vi "WhoInheritsWhom.vi"(0 "reference":refnum<class "ClassRelationshipEdge.lvclass">, 5 "error in (no error)":errorcluster) -> (14 "reference out":refnum<class "ClassRelationshipEdge.lvclass">, 15 "inherits":refnum<class "AbstractNode.lvclass">, 16 "base":refnum<class "AbstractNode.lvclass">, 17 "inheritanceUsed":bool, 19 "error out":errorcluster)   [LabVIEW 2016, in "ClassRelationshipEdge.lvclass"]
doc: "In which direction is the Triangle point, pointing."
uses:
  <resource>/Framework/Providers/Open_GDS/UML/ClassRelationshipEdge_class/ClassRelationshipEdge.lvclass
  C:/Program Files (x86)/National Instruments/LabVIEW 2016/resource/Framework/Providers/Open_GDS/UML/SegmentedLineEdge_class/SegmentedLineEdge.lvclass
  C:/Program Files (x86)/National Instruments/LabVIEW 2016/resource/Framework/Providers/Open_GDS/UML/AbstractEdge_class/AbstractEdge.lvclass
  <resource>/Framework/Providers/Open_GDS/UML/AbstractNode_class/AbstractNode.lvclass
  <resource>/Framework/Providers/Open_GDS/UML/ArrowHead_class/ArrowHead.lvclass
  <resource>/Framework/Providers/Open_GDS/UML/SegmentedLineEdge_class/SegmentedLineEdge.lvclass
  <resource>/Framework/Providers/Open_GDS/UML/AbstractEdge_class/AbstractEdge.lvclass
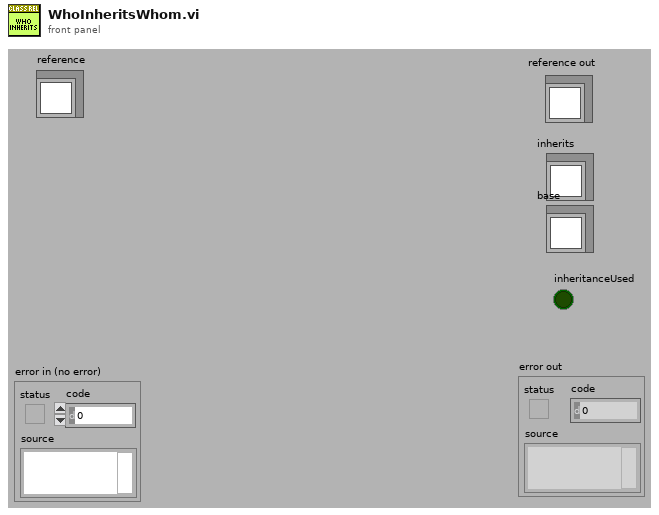
[diagram p1: front panel]
types:
  T1 = typedef "SegmentedLineEdge.lvclass/ObjectAttributes.ctl" = cluster{"lineStyle":refnum<class "LineStyle.lvclass">, "startArrowHead":refnum<class "ArrowHead.lvclass">, "endArrowHead":refnum<class "ArrowHead.lvclass">, "startLabel":string, "midLabel":string, "endLabel":string, "MidLabelOffset":T2, "SplitWire":bool}
  T2 = typedef "Point Point2D.ctl" = cluster{"x":dbl, "y":dbl}
  T3 = typedef "AbstractEdge.lvclass/ObjectAttributes.ctl" = cluster{"start":refnum<class "AbstractNode.lvclass">, "end":refnum<class "AbstractNode.lvclass">}
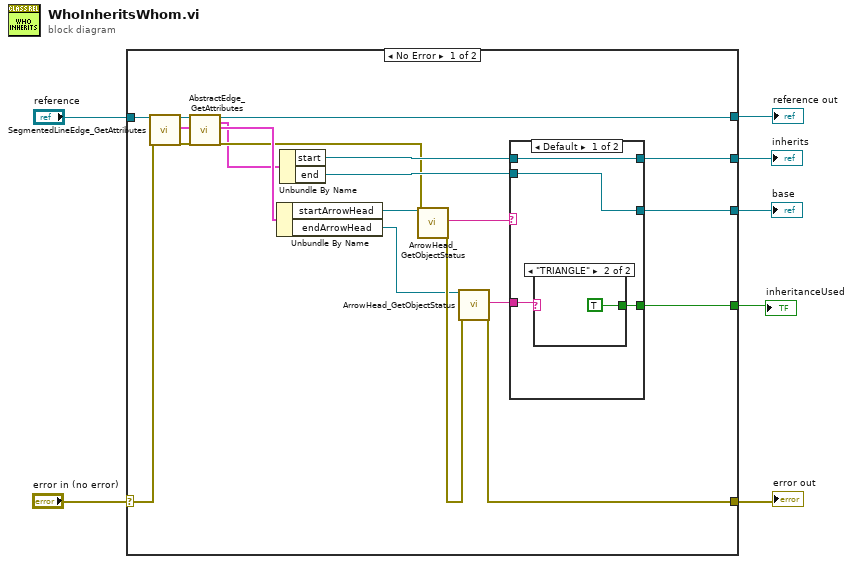
[diagram p0: block diagram]
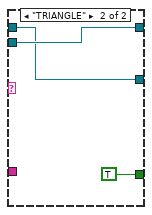
[diagram p3: hidden frame]
diagram:
  n1 = case shown="No Error" "error in (no error)" {
    selector: "error in (no error)" -> [w26 w35]
    tunnel: "reference" -> [w25 w36]
    tunnel: [w18 w35] -> w5
    tunnel: [w11 w36] -> w4
    tunnel: [w21 _] -> w3
    tunnel: [w20 _] -> w2
    tunnel: [w16 _] -> w1
    frame No Error {
      n2 = call <resource>:"SegmentedLineEdge_GetAttributes.vi"("reference in"=w25, "error in (no error)"=w26) -> ("reference out"=w14:refnum<class "ClassRelationshipEdge.lvclass">, "Data"=w15:T1, "error out"=w13:errorcluster)  [unwired: 14 in, 1 out]
      n3 = call <resource>:"AbstractEdge_GetAttributes.vi"("reference in"=w14, "error in (no error)"=w13) -> ("reference out"=w11:refnum<class "ClassRelationshipEdge.lvclass">, "Data"=w10:T3, "error out"=w12:errorcluster)  [unwired: 14 in, 1 out]
      n4 = Unbundle By Name(w15) -> ("startArrowHead"=w24:refnum<class "ArrowHead.lvclass">, "endArrowHead"=w17:refnum<class "ArrowHead.lvclass">)
      n5 = Unbundle By Name(w10) -> ("start"=w23:refnum<class "AbstractNode.lvclass">, "end"=w22:refnum<class "AbstractNode.lvclass">)
      n6 = call <resource>:"ArrowHead_GetObjectStatus.vi"("reference in"=w24, "error in (no error)"=w12) -> ("Object name"=w9:string, "error out"=w19:errorcluster)  [unwired: 1 in, 15 out]
      n7 = call <resource>:"ArrowHead_GetObjectStatus.vi"("reference in"=w17, "error in (no error)"=w19) -> ("Object name"=w8:string, "error out"=w18:errorcluster)  [unwired: 1 in, 15 out]
      n8 = case shown="Default" w9 {
        tunnel: w23 -> [w30 w33]
        tunnel: w22 -> [w29 w34]
        tunnel: [w30 w34] -> w21
        tunnel: [w29 w33] -> w20
        tunnel: w8 -> [w28 _]
        tunnel: [w27 TRUE] -> w16
        frame Default {
          n9 = case shown="\"TRIANGLE\"" w28 {
            tunnel: [_ TRUE] -> w27
            frame Default {
            }
            frame "TRIANGLE" {
            }
          }
        }
        frame "TRIANGLE" {
        }
      }
    }
    frame Error {
    }
  }
  "reference out" <- w4
  "error out" <- w5
  "inherits" <- w3
  "base" <- w2
  "inheritanceUsed" <- w1
